vi "PhaseImbDemo.vi"() -> ()   [LabVIEW 2009]
uses:
  <vilib>/imath/engines/lvmath2/RunTimeEngine/ErrorHandling/NIMS_Finalize Error.vi
  <vilib>/imath/engines/lvmath2/RunTimeEngine/Parser/MC_Version.vi
  <vilib>/imathl/engines/lvmath/Functions/Error Handling/Create Error.vi
  <vilib>/imath/engines/lvmath2/RunTimeEngine/BuiltInFunctions/zeros/NIMS_M=zeros(I32,I32).vi
  <vilib>/imath/engines/lvmath2/RunTimeEngine/NodeEndStatement/NIMS_NodeEndStatement_Output.vi
  <instcachedir>/0/NIMS_NodeEndStatement_Output_53EC0D466D134D7ABD903AC30B43404B.lvgen/NIMS_NodeEndStatement_Output_53EC0D466D134D7ABD903AC30B43404B_001.vi
  <instcachedir>/0/NIMS_NodeEndStatement_Output_53EC0D466D134D7ABD903AC30B43404B.lvgen/NIMS_NodeEndStatement_Output_53EC0D466D134D7ABD903AC30B43404B_000.vi
  <vilib>/imath/engines/lvmath2/RunTimeEngine/RangeToken/NIMS_Range.vi
  <instcachedir>/0/NIMS_Range_08574DECC23E450FAF0AC0BC39E6BEA7.lvgen/NIMS_Range_08574DECC23E450FAF0AC0BC39E6BEA7_001.vi
  <vilib>/imath/engines/lvmath2/RunTimeEngine/ArithmeticOperatorToken/NIMS_ArithmeticOperator_plus.vi
  <instcachedir>/0/NIMS_ArithmeticOperator_plus_48B9519178ED42D7840F01273E784BFE.lvgen/NIMS_ArithmeticOperator_plus_48B9519178ED42D7840F01273E784BFE_001.vi
  <vilib>/imath/engines/lvmath/Functions/Error Handling/MergeErrorsWrapper.vi
  <vilib>/imath/engines/lvmath/Functions/Error Handling/MC_Error Cluster From Error Code.vi
  <vilib>/imath/engines/lvmath2/RunTimeEngine/BuiltInFunctions/fft/NIMS_fft(GV).vi
  <instcachedir>/0/NIMS_fft(GV)_4C6467FC22F84E4BA42517A07EF978B0.lvgen/NIMS_fft(GV)_4C6467FC22F84E4BA42517A07EF978B0_000.vi
  <vilib>/imath/engines/lvmath2/RunTimeEngine/BuiltInFunctions/abs/NIMS_abs(signed).vi
  <instcachedir>/0/NIMS_abs(signed)_C4FCB8E6058B49B797C7C8D53CA5F6EC.lvgen/NIMS_abs(signed)_C4FCB8E6058B49B797C7C8D53CA5F6EC_000.vi
  <vilib>/imath/engines/lvmath/Plug In/_Char/NIMS_CH_character datatype.ctl
  <vilib>/imath/engines/lvmath/Plug In/_Char/NIMS_CH_String to Character Array.vi
  <vilib>/imath/engines/lvmath2/RunTimeEngine/BuiltInFunctions/sprintf/NIMS_sprintf(Str,RS,RS).vi
  <vilib>/imath/engines/lvmath2/RunTimeEngine/VariableToken/Read/NIMS_Get Elements - RV(_) - Check(_).vi
  <instcachedir>/0/NIMS_Get Elements - RV(_) - Check(_)_FD08F12CA9A340B3A4DC1D5FF02404A0.lvgen/NIMS_Get Elements - RV(_) - Check(_)_FD08F12CA9A340B3A4DC1D5FF02404A0_001.vi
  <vilib>/imath/engines/lvmath/Plug In/_Char/NIMS_CH_Character RV to String.vi
  <instcachedir>/0/NIMS_Get Elements - RV(_) - Check(_)_FD08F12CA9A340B3A4DC1D5FF02404A0.lvgen/NIMS_Get Elements - RV(_) - Check(_)_FD08F12CA9A340B3A4DC1D5FF02404A0_002.vi
  <vilib>/imath/engines/lvmath2/RunTimeEngine/BuiltInFunctions/sprintf/NIMS_sprintf(Str,RM).vi
panel:
  out "Phase Imbalance (degrees)":dbl
  out "pwrImbal (dB)":dbl
  out "pwrTotdB (dB)":dbl
  out "pwrTot (W)":dbl
  out "Result2db (dB)":dbl
  out "Resultdb (dB)":dbl
  out "Result2 (V)":dbl
  out "Result (V)":dbl
  out "Power2 (W)":dbl
  out "Power (W)":dbl
  out "Bin2":dbl
  out "Bin1":dbl
  out "error out":errorcluster
  in  "Next":bool
  in  "Number of Iterations":u8=5
  out "Power dB":dbl[](graph)
  in  "As":dbl=1.0
  in  "Ac":dbl=1.0
  in  "M":dbl=10.0
  in  "N":dbl=64.0
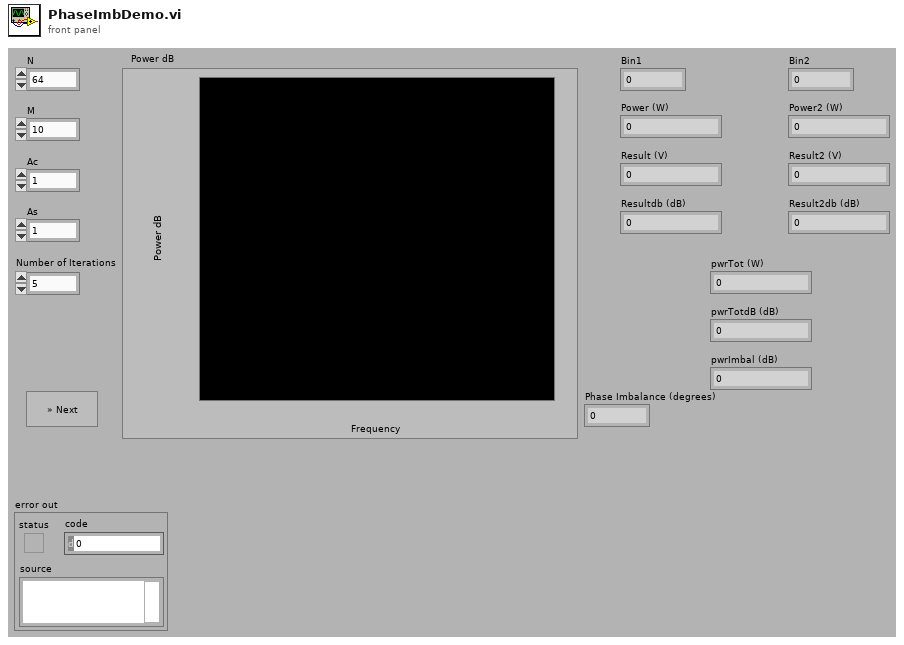
[diagram p1: front panel]
types:
  T1 = cluster{"Numeric 2":dbl, "Numeric 3":dbl, "Numeric 4":dbl}
  T2 = typedef "NIMS_CH_character datatype.ctl" = cluster{"Numeric":u8}
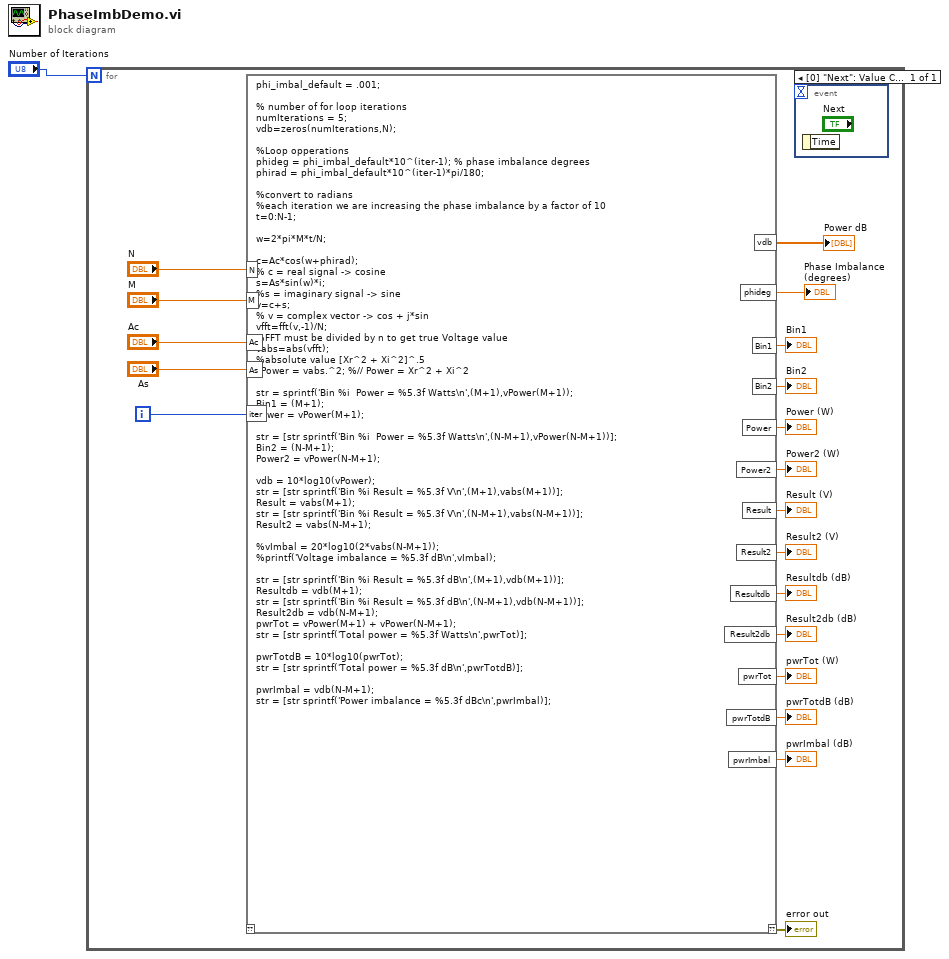
[diagram p0: block diagram]
diagram:
  n1 = for {
    N: "Number of Iterations" -> [_]
    i -> [w14]
    n2 = mathscript code="phi_imbal_default = .001;\n\n% number of for loop iterations\nnumIterations = 5;\nvdb=zeros(numIterations,N);\n\n%Loop opperations\nphideg = phi_imbal_default*10^(iter-1); % phase imbalance degrees\nphirad = phi_imbal_default*10^(iter-1)*pi/180;\n\n%convert to radians\n%each iteration we are increasing the phase imbalance by a factor of 10\nt=0:N-1;\n\nw=2*pi*M*t/N;\n\nc=Ac*cos(w+phirad);\n% c = real signal -> cosine\ns=As*sin(w)*i;\n%s = imaginary signal -> sine\nv=c+s; \n% v = complex vector -> cos + j*sin\nvfft=fft(v,-1)/N;\n%FFT must be divided by n to get true Voltage value\nvabs=abs(vfft);\n%absolute value [Xr^2 + Xi^2]^.5\nvPower = vabs.^2; %// Power = Xr^2 + Xi^2\n\nstr = sprintf('Bin %i  Power = %5.3f Watts\\n',(M+1),vPower(M+1));\nBin1 = (M+1);\nPower = vPower(M+1);\n\nstr = [str sprintf('Bin %i  Power = %5.3f Watts\\n',(N-M+1),vPower(N-M+1))];\nBin2 = (N-M+1);\nPower2 = vPower(N-M+1);\n\nvdb = 10*log10(vPower);\nstr = [str sprintf('Bin %i Result = %5.3f V\\n',(M+1),vabs(M+1))];\nResult = vabs(M+1);\nstr = [str sprintf('Bin %i Result = %5.3f V\\n',(N-M+1),vabs(N-M+1))];\nResult2 = vabs(N-M+1);\n\n%vImbal = 20*log10(2*vabs(N-M+1));\n%printf('Voltage imbalance = %5.3f dB\\n',vImbal);\n\nstr = [str sprintf('Bin %i Result = %5.3f dB\\n',(M+1),vdb(M+1))];\nResultdb = vdb(M+1);\nstr = [str sprintf('Bin %i Result = %5.3f dB\\n',(N-M+1),vdb(N-M+1))];\nResult2db = vdb(N-M+1);\npwrTot = vPower(M+1) + vPower(N-M+1);\nstr = [str sprintf('Total power = %5.3f Watts\\n',pwrTot)];\n\npwrTotdB = 10*log10(pwrTot);\nstr = [str sprintf('Total power = %5.3f dB\\n',pwrTotdB)];\n\npwrImbal = vdb(N-M+1);\nstr = [str sprintf('Power imbalance = %5.3f dBc\\n',pwrImbal)];"("N"="N", "M"="M", "Ac"="Ac", "As"="As", "iter"=w14) -> ("??"=→"error out":errorcluster, "vdb"=→"Power dB":dbl[], "Bin1"=→"Bin1":dbl, "Bin2"=→"Bin2":dbl, "Power"=→"Power (W)":dbl, "Power2"=→"Power2 (W)":dbl, "Result"=→"Result (V)":dbl, "Result2"=→"Result2 (V)":dbl, "Resultdb"=→"Resultdb (dB)":dbl, "Result2db"=→"Result2db (dB)":dbl, "pwrTot"=→"pwrTot (W)":dbl, "pwrTotdB"=→"pwrTotdB (dB)":dbl, "pwrImbal"=→"pwrImbal (dB)":dbl, "phideg"=→"Phase Imbalance (degrees)":dbl)  [unwired: 1 in]
    n3 = event shown="[0] \"Next\": Value Change" {
      selector: _ -> [_]
      dyn-events: _ -> [_]
      timeout: _ -> [_]
      event [0] "Next": Value Change {
        n4 = event-data() -> ()  [unwired: 1 in, 1 out]
      }
    }
  }
